vi "oa_Auto Scale for SCL Plot.vi"(8 "error in (no error)":errorcluster, 10 "scale in":T1, 11 "DC Gap":cluster{"X":dbl[], "Y":dbl[]}[](array[cluster]) {"Y" format="%.2f"; "X" format="%.2f"}) -> (0 "error out":errorcluster, 2 "scale":T1, 3 "DC Gap out":cluster{"X":dbl[], "Y":dbl[]}[](array[cluster]) {"Y" format="%.2f"; "X" format="%.2f"})   [LabVIEW 2017]
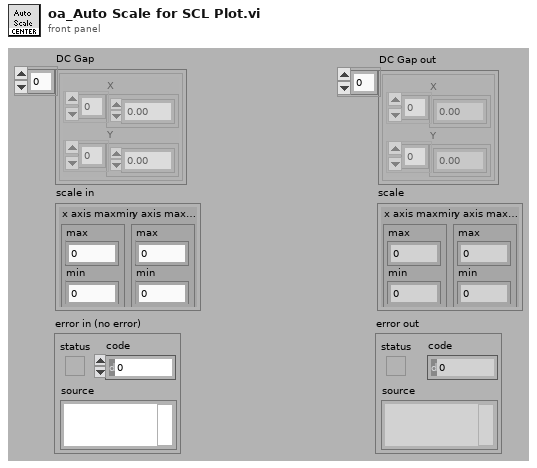
[diagram p1: front panel]
types:
  T1 = cluster{"x axis maxmin":cluster{"max":dbl, "min":dbl}, "y axis maxmin":cluster{"max":dbl, "min":dbl}}
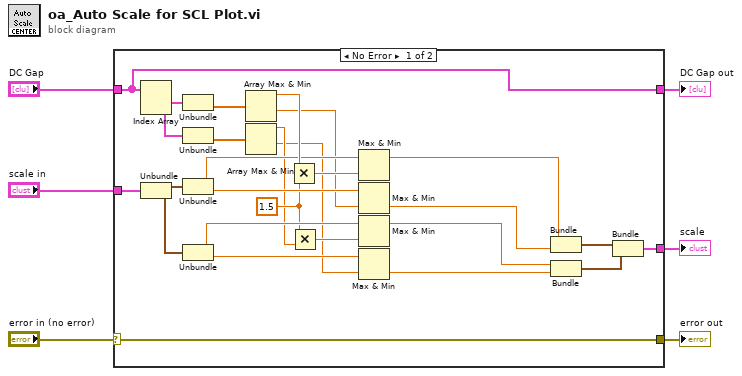
[diagram p0: block diagram]
diagram:
  n1 = case shown="No Error" "error in (no error)" {
    selector: "error in (no error)" -> [w30 w36]
    tunnel: [w30 w36] -> w5
    tunnel: "DC Gap" -> [w29 w35]
    tunnel: [w31 w34] -> w3
    tunnel: [w29 w35] -> w2
    tunnel: "scale in" -> [w28 w34]
    frame No Error {
      w18 = 1.5 ("y")
      n2 = Index Array(array=w29) -> (element #1=w33:cluster{"X":dbl[], "Y":dbl[]}, element #2=w32:cluster{"X":dbl[], "Y":dbl[]})  [unwired: 2 in]
      n3 = Unbundle(w28) -> ("x axis maxmin"=w26:cluster{"max":dbl, "min":dbl}, "y axis maxmin"=w25:cluster{"max":dbl, "min":dbl})
      n4 = Unbundle(w33) -> ("Y"=w15:dbl[])  [unwired: 1 out]
      n5 = Unbundle(w32) -> ("Y"=w14:dbl[])  [unwired: 1 out]
      n6 = Unbundle(w26) -> ("max"=w24:dbl, "min"=w22:dbl)
      n7 = Unbundle(w25) -> ("max"=w21:dbl, "min"=w19:dbl)
      n8 = Array Max & Min(array=w15) -> (max value=w27:dbl, min value=w13:dbl)  [unwired: 2 out]
      n9 = Array Max & Min(array=w14) -> (max value=w17:dbl, min value=w12:dbl)  [unwired: 2 out]
      n10 = Multiply(x=w27, y=w18) -> (x*y=w23:dbl)
      n11 = Multiply(x=w18, y=w17) -> (x*y=w20:dbl)
      n12 = Max & Min(x=w24, y=w23) -> (max(x,y)=w11:dbl)  [unwired: 1 out]
      n13 = Max & Min(x=w22, y=w13) -> (min(x,y)=w10:dbl)  [unwired: 1 out]
      n14 = Max & Min(x=w21, y=w20) -> (max(x,y)=w9:dbl)  [unwired: 1 out]
      n15 = Max & Min(x=w19, y=w12) -> (min(x,y)=w8:dbl)  [unwired: 1 out]
      n16 = Bundle(w11, w10) -> (w16:cluster{dbl, dbl})  [unwired: 1 in]
      n17 = Bundle(w9, w8) -> (w7:cluster{dbl, dbl})  [unwired: 1 in]
      n18 = Bundle(w16, w7) -> (w31:cluster{cluster{dbl, dbl}, cluster{dbl, dbl}})  [unwired: 1 in]
    }
    frame Error {
    }
  }
  "error out" <- w5
  "DC Gap out" <- w2
  "scale" <- w3
